vi "Configure SLSC Switch Custom Device.vi"(6 "product name":string, 8 "error in":errorcluster, 9 "switches json":string, 10 "topologies":string[](array[string]), 11 "slsc switch custom device in":T1 format="%.0x") -> (0 "error out":errorcluster, 3 "slsc switch custom device out":T1 format="%.0x")   [LabVIEW 2020, in "SLSC Switch Scripting.lvlib"]
uses:
  SLSC Switch Scripting.lvlib
  <vilib>/NI VeriStand/Custom Device API/Custom Device Item Ref.ctl
  Properties/SLSC Switch All Properties.ctl
  <vilib>/NI VeriStand/Custom Device API/Custom Device API.lvlib
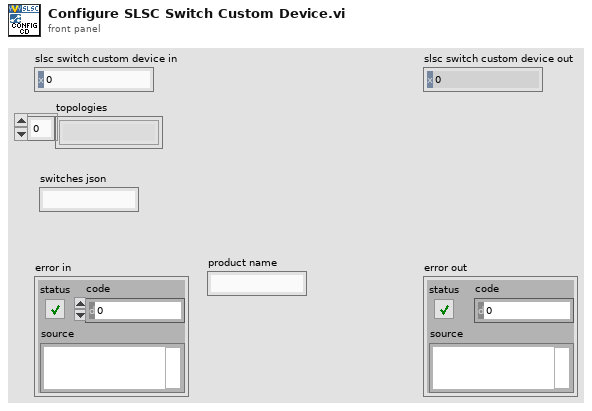
[diagram p1: front panel]
types:
  T1 = typedef "Custom Device API.lvlib/Custom Device Item Ref.ctl" = u64
  T2 = typedef "SLSC Switch Scripting.lvlib/SLSC Switch All Properties.ctl" = cluster{"Product Name":string, "Topology":string, "Switches JSON":string, "Description":string, "Reservation Group":string}
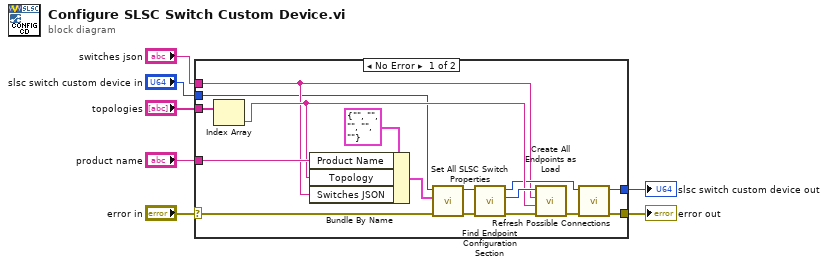
[diagram p0: block diagram]
diagram:
  n1 = case shown="No Error" "error in" {
    selector: "error in" -> [w10 w24]
    tunnel: "product name" -> [w23 _]
    tunnel: [w8 w24] -> w6
    tunnel: [w9 w25] -> w5
    tunnel: "topologies" -> [w13 _]
    tunnel: "switches json" -> [w12 _]
    tunnel: "slsc switch custom device in" -> [w11 w25]
    frame No Error {
      n2 = Index Array(array=w13) -> (element=w19:string)  [unwired: 1 in]
      n3 = Bundle By Name(cluster=T2 {"Product Name"="", "Topology"="", "Switches JSON"="", "Description"="", "Reservation Group"=""} ("SLSC Switch All Properties"), "Product Name"=w23, "Topology"=w19, "Switches JSON"=w12) -> (w14:T2)
      n4 = call "Set All SLSC Switch Properties.vi"("error in"=w10, "properties"=w14, "slsc switch custom device in"=w11) -> ("error out"=w22:errorcluster, "slsc switch custom device out"=w16:T1)  [unwired: 7 in]
      n5 = call "Find Endpoint Configuration Section.vi"("error in"=w22, "slsc switch custom device in"=w16) -> ("error out"=w21:errorcluster, "endpoint configuration"=w20:T1, "slsc switch custom device out"=w18:T1)  [unwired: 7 in]
      n6 = call "Create All Endpoints as Load.vi"("error in"=w21, "topology"=w19, "switches json"=w12, "endpoint configuration in"=w20) -> ("error out"=w17:errorcluster)  [unwired: 6 in, 1 out]
      n7 = call "Refresh Possible Connections.vi"("error in"=w17, "slsc switch custom device in"=w18) -> ("error out"=w8:errorcluster, "slsc switch custom device out"=w9:T1)  [unwired: 8 in]
    }
    frame Error {
    }
  }
  "error out" <- w6
  "slsc switch custom device out" <- w5
